vi "Get Style.vi"(8 "error in (no error)":errorcluster, 11 "Graphic in":refnum<class "Graphic.lvclass">) -> (0 "error out":errorcluster, 2 "Style":T1={"Color"=0, "Pen"={"Width"=2, "Style"=enum."Solid"}}, 3 "Graphic out":refnum<class "Graphic.lvclass">)   [LabVIEW 2015, in "Graphic.lvclass"]
uses:
  Graphic.lvclass
  Ctls/Style.ctl
  Graphic.lvclass/Graphic.ctl
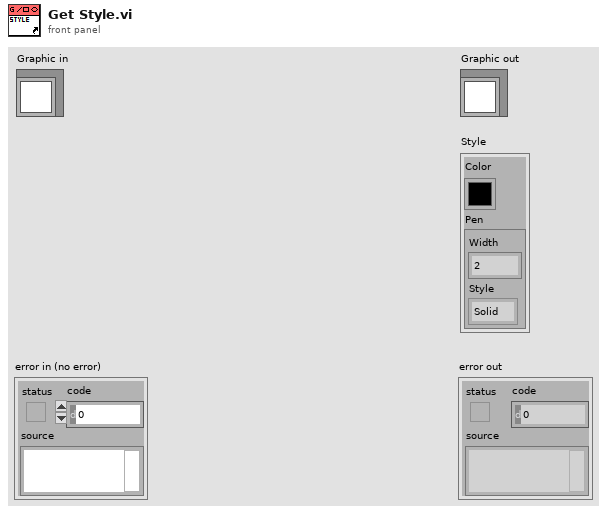
[diagram p1: front panel]
types:
  T1 = typedef "Graphic.lvclass/Style.ctl" = cluster{"Color":u32, "Pen":cluster{"Width":u16, "Style":enum32{"Solid", "Dash", "Dot", "DashDot", "DashDotDot"}}}
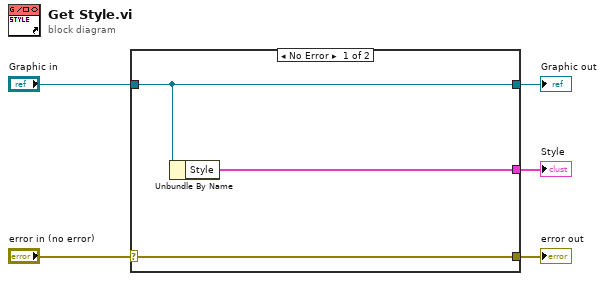
[diagram p0: block diagram]
diagram:
  n1 = case shown="No Error" "error in (no error)" {
    selector: "error in (no error)" -> [w8 w9]
    tunnel: [w8 w9] -> w4
    tunnel: [w7 w10] -> w2
    tunnel: "Graphic in" -> [w7 w10]
    tunnel: [w6 _] -> w1
    frame No Error {
      n2 = Unbundle By Name(w7) -> ("Style"=w6:T1)
    }
    frame Error {
    }
  }
  "error out" <- w4
  "Graphic out" <- w2
  "Style" <- w1
